vi "VI to JSON Graph Descr.vi"(8 "error in (no error)":errorcluster, 11 "vi path":path) -> (0 "error out":errorcluster, 2 "VI Description":string, 3 "JSON VI Graph":string)   [LabVIEW 2020]
doc: "**vi to json graph descrp.vi** scans recursivly a VI's Block Diagram\n(including nested structures such as Loops and Case Structures) and returns a JSON object describing all objects, their wiring, and constant values. Output has four top-level array keys:\n\n\"0\" — Objects\n Every GObject found on the diagram: nodes, terminals, wires, diagrams,\n structures, constants.\n Fields: ClassID (LabVIEW internal class ID), UID (unique ref ID, valid\n for this scan only), ClassName (e.g. \"Function\", \"Wire\", \"Terminal\",\n \"ForLoop\", \"DigitalNumericConstant\"), LabelText (visible caption, if\n any), OwnerClass / OwnerName / Ownder_UID (immediate parent GObject).\n Note: \"Ownder_UID\" is a known typo in the field name, kept as-is for\n compatibility — do not treat it as an error.\n\n\"1\" — Wires (node-level)\n One entry per wire. UID_Wire (matches a \"Wire\" Object in array 0),\n UID_Source (owning-node UID of the wire's source terminal), UIDs_Sink\n (owning-node UID(s) of its sink terminal(s)). A wire may branch to\n multiple sinks; the same node UID can appear more than once if several\n of its terminals are fed by the same wire.\n\n\"2\" — Terminal-Wire mapping\n Resolves array \"1\" down to the exact terminal. Fields: \"Terminal UID\"\n (matches a Terminal-class Object in array 0), \"Wire UID\", \"Caption\"\n (the terminal's visible name/role, e.g. \"x\", \"output cluster\", \"x+1\";\n empty if the terminal has no visible caption).\n\n\"3\" — Constant values\n Fields: \"Constant UID\" (matches a *Constant-class Object in array 0),\n \"Value String\" (the constant's value as a JSON-formatted string). For\n ClusterConstant this is a full nested JSON object of all its fields.\n\nResolving a wire to its exact source/sink terminals:\n 1. Look up the wire in array \"1\" ? UID_Source, UIDs_Sink (node-level).\n 2. Find all entries in array \"2\" with matching \"Wire UID\" ? candidate\n terminal UIDs.\n 3. For each candidate, look up its Ownder_UID in array \"0\": if it\n equals UID_Source, that terminal is the source; if it appears in\n UIDs_Sink, it is a sink terminal.\n 4. Use \"Caption\" from array \"2\" for the terminal's semantic role\n (cluster field name, parameter name, etc.).\n\nKnown limitations:\n - Duplicate object entries may occasionally appear for the same UID\n (root cause not yet identified).\n - ClusterConstant \"Value String\" duplicates the values of its child\n constants (also listed individually) — provided as a convenience\n aggregate, not an independent value.\n - A constant's LabelText is a free-form caption; it is not necessarily\n related to the terminal/field it feeds."
uses:
  <vilib>/Utility/traverseref.llb/TRef TravTarget.ctl
  ObjDescription.ctl
  Value of Constant.ctl
  Terminal and Wire.ctl
  Wire_Source_and_Sinks_IDs.ctl
  <vilib>/Utility/traverseref.llb/VI Scripting - Traverse.lvlib
  <vilib>/JDP Science/JSONtext/JSONtext.lvlib
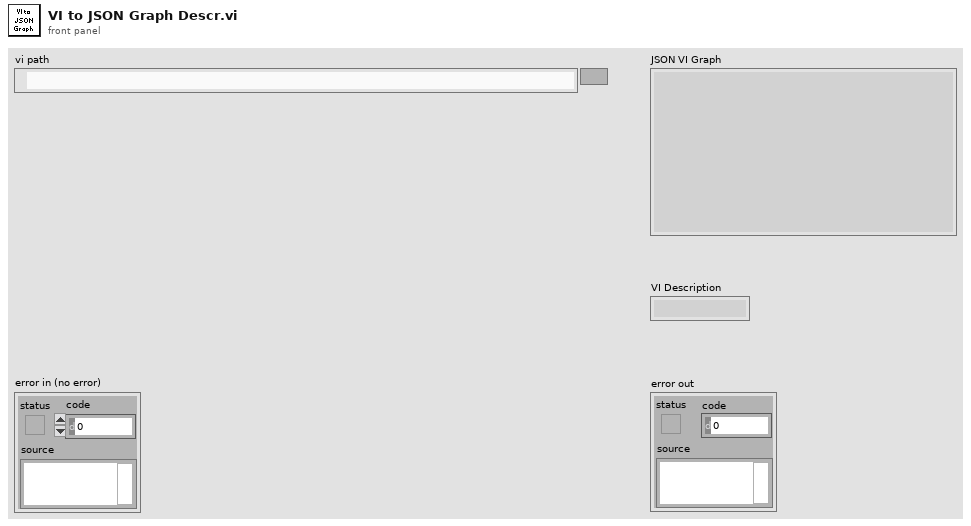
[diagram p1: front panel]
types:
  T1 = typedef "TRef TravTarget.ctl" = enum16{"FP", "BD", "Other"}
  T2 = typedef "ObjDescription.ctl" = cluster{"ClassID":u32, "UID":u32, "ClassName":string, "LabelText":string, "OwnerClass":string, "OwnerName":string, "Ownder_UID":u32}
  T3 = typedef "Value of Constant.ctl" = cluster{"Constant UID":i32, "Value String":string}
  T4 = typedef "Wire_Source_and_Sinks_IDs.ctl" = cluster{"UID_Wire":i32, "UID_Source":i32, "UIDs_Sink":i32[]}
  T5 = typedef "Terminal and Wire.ctl" = cluster{"Terminal UID":i32, "Wire UID":i32, "Caption":string}
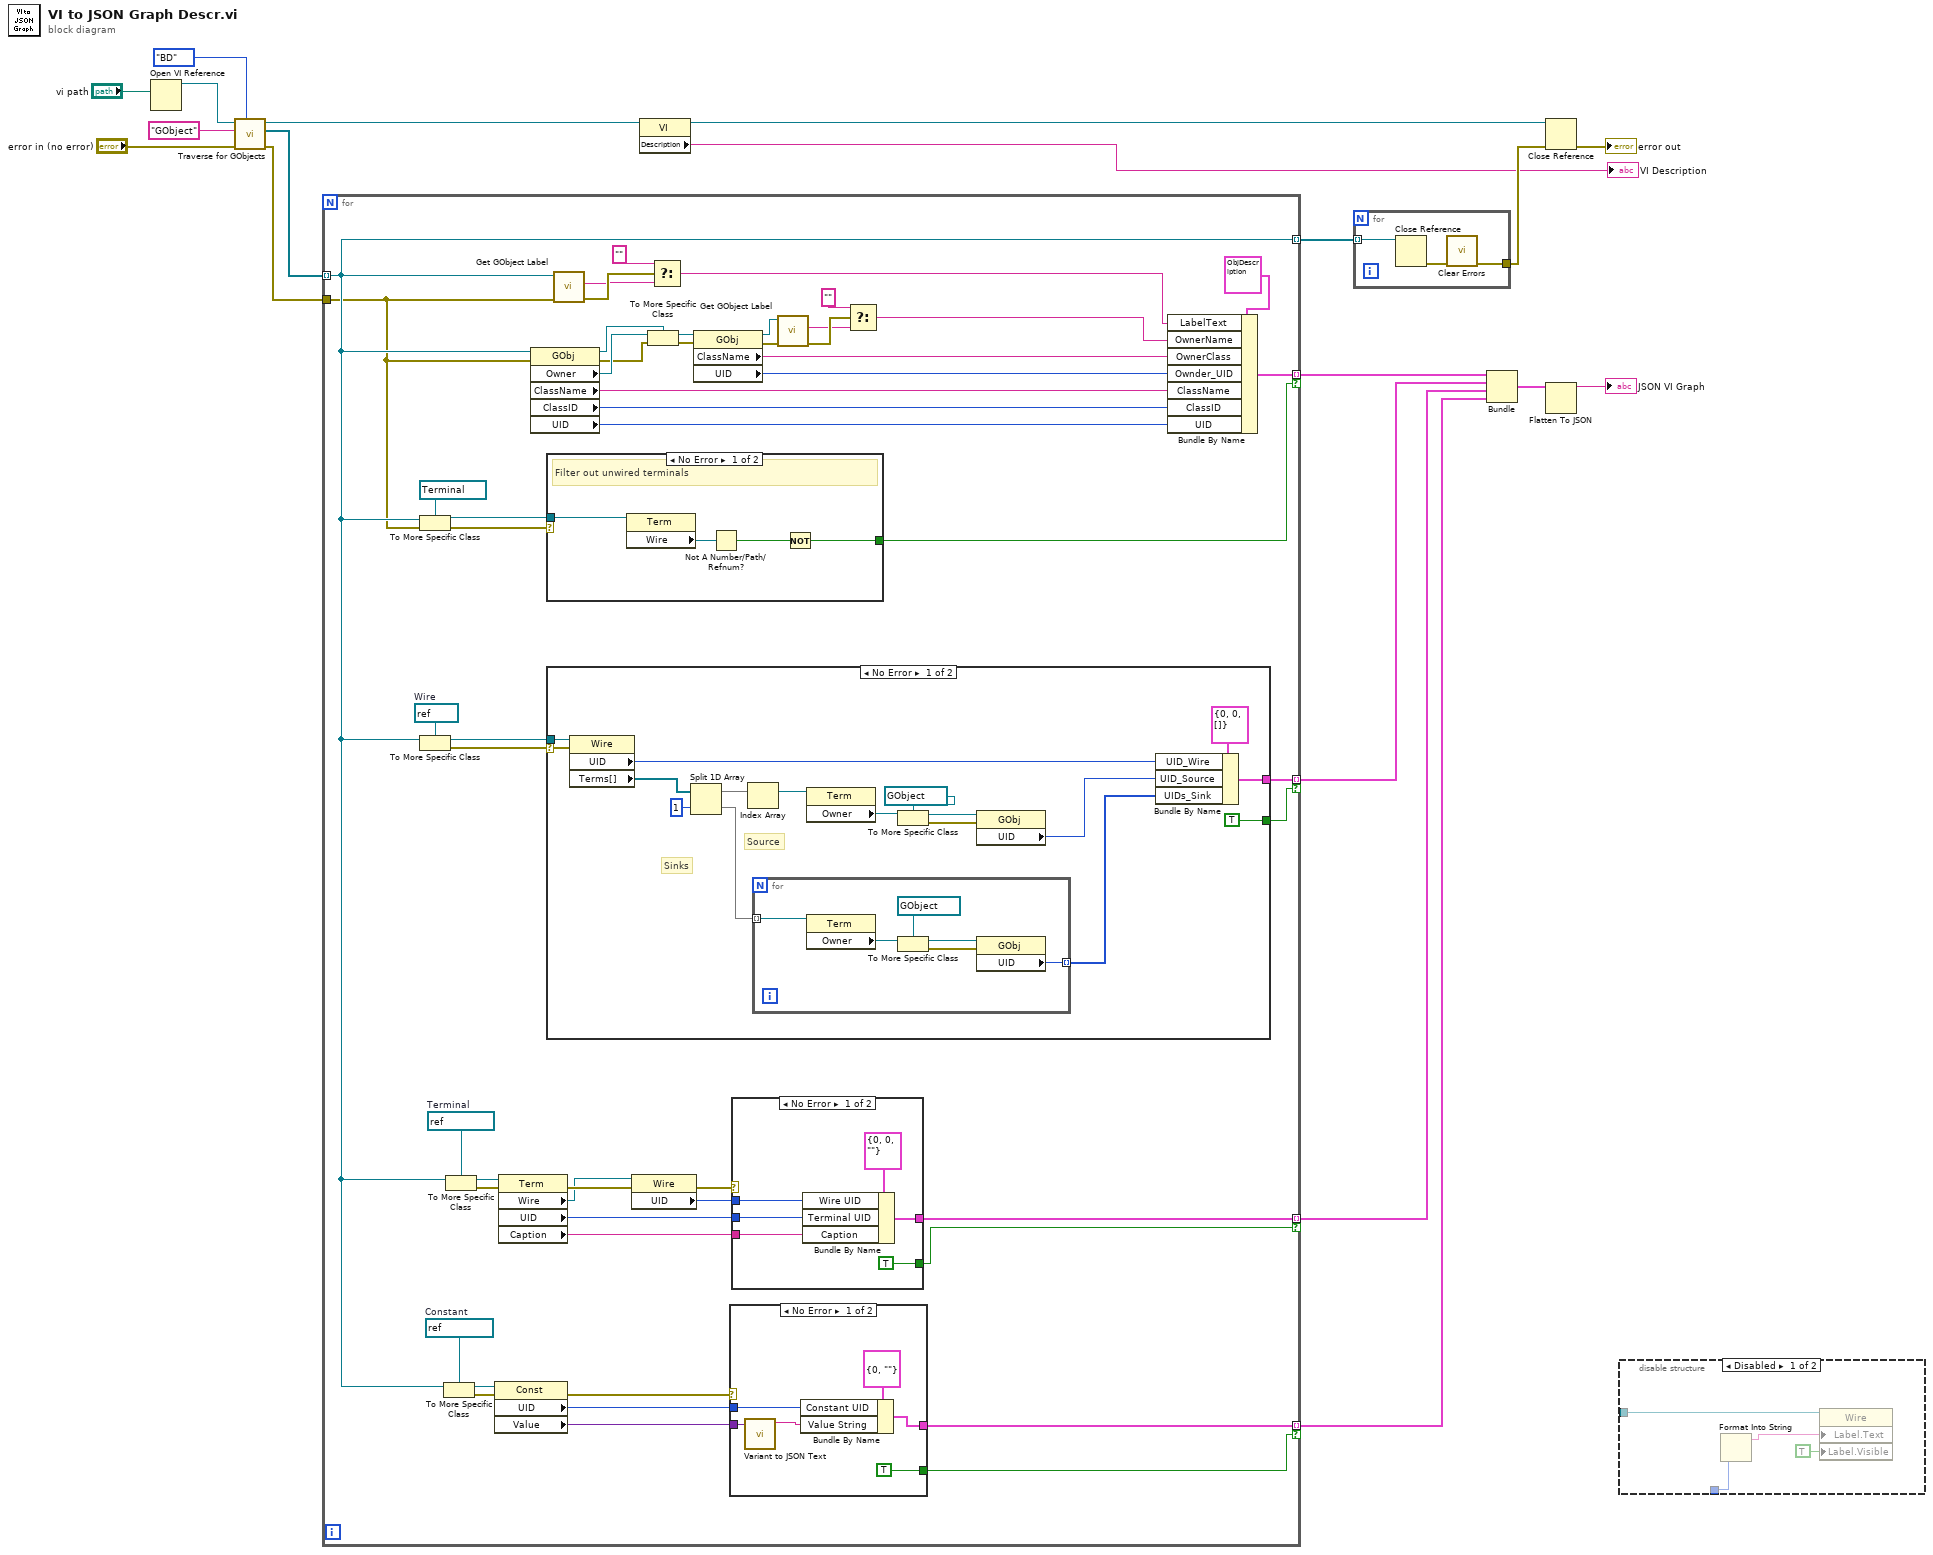
[diagram p0: block diagram]
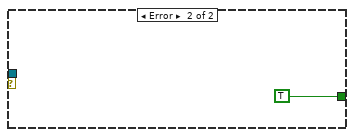
[diagram p2: hidden frame]
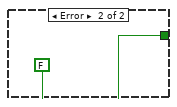
[diagram p4: hidden frame]
diagram:
  n1 = Open VI Reference(vi path="vi path") -> (vi reference=w17:refnum<vi>)  [unwired: 5 in, 1 out]
  n2 = call <vilib>:"Traverse for GObjects.vi"("Traverse Target"=TRef_TravTarget."BD", "error in (no error)"="error in (no error)", "Class Name"="GObject", "VI Refnum"=w17) -> ("error out"=w12:errorcluster, "References"=w19:refnum<vi>[], "dup VI Refnum"=w3:refnum<vi>)  [unwired: 4 in, 1 out]
  n3 = for {
    tunnel: w19 -> [w25] mode=indexing
    tunnel: [w66] -> w8 mode=indexing if=w20
    tunnel: [w25] -> w13 mode=indexing
    tunnel: w12 -> [w22]
    tunnel: [w46] -> w9 mode=indexing if=w45
    tunnel: [w43] -> w6 mode=indexing if=w42
    tunnel: [w27] -> w4 mode=indexing if=w26
    w30 = refnum<vi> refnum  # Constant
    w44 = refnum<vi> refnum  # Terminal
    w52 = refnum<vi> refnum  # Wire
    n4 = To More Specific Class(target class=refnum<vi> refnum ("reference out"), reference=w25, error in=w22) -> (specific class reference=w23:refnum<vi>, error out=w21:errorcluster)
    n5 = To More Specific Class(target class=w52, reference=w25) -> (specific class reference=w51:refnum<vi>, error out=w50:errorcluster)  [unwired: 1 in]
    n6 = To More Specific Class(target class=w30, reference=w25) -> (specific class reference=w31:refnum<vi>, error out=w32:errorcluster)  [unwired: 1 in]
    n7 = To More Specific Class(target class=w44, reference=w25) -> (specific class reference=w41:refnum<vi>, error out=w39:errorcluster)  [unwired: 1 in]
    n8 = property class="Const"(reference=w31, error in=w32) -> (error out=w33:errorcluster, "UID"=w28:i32, "Value"=w29:variant)  [unwired: 1 out]
    n9 = property class="Term"(reference=w41, error in=w39) -> (error out=w38:errorcluster, "Wire"=w35:refnum<vi>, "UID"=w34:i32, "Caption"=w36:string)  [unwired: 1 out]
    n10 = property class="GObj"(reference=w25, error in=w22) -> (reference out=w53:refnum<vi>, error out=w57:errorcluster, "Owner"=w69:refnum<vi>, "ClassName"=w48:string, "ClassID"=w47:u32, "UID"=w55:i32)
    n11 = case shown="No Error" w21 {
      tunnel: w23 -> [w75 _]
      tunnel: [w72 TRUE] -> w20
      frame No Error {
        # "Filter out unwired terminals"
        n12 = property class="Term"(reference=w75) -> ("Wire"=w74:refnum<vi>)  [unwired: 1 in, 2 out]
        n13 = Not A Number/Path/Refnum?(number/path/refnum=w74) -> (NaN/Path/Refnum?=w73:bool)
        n14 = Not(x=w73) -> (.not. x?=w72:bool)
      }
      frame Error {
      }
    }
    n15 = case shown="No Error" w50 {
      selector: w50 -> [w98 _]
      tunnel: w51 -> [w99 _]
      tunnel: [w89 _] -> w46
      tunnel: [TRUE FALSE] -> w45
      frame No Error {
        # "Sinks"
        # "Source"
        n16 = property class="Wire"(reference=w99, error in=w98) -> ("UID"=w83:i32, "Terms[]"=w87:refnum<vi>[])  [unwired: 2 out]
        n17 = Split 1D Array(array=w87, index=1 ("length")) -> (first subarray=w95:refnum<vi>[], second subarray=w94:refnum<vi>[])
        n18 = Index Array(array=w95) -> (element=w96:refnum<vi>)  [unwired: 1 in]
        n19 = for {
          tunnel: w94 -> [w105] mode=indexing
          tunnel: [w100] -> w84 mode=indexing
          n20 = property class="Term"(reference=w105) -> ("Owner"=w101:refnum<vi>)  [unwired: 1 in, 2 out]
          n21 = To More Specific Class(target class=refnum<vi> refnum ("reference out"), reference=w101) -> (specific class reference=w103:refnum<vi>, error out=w102:errorcluster)  [unwired: 1 in]
          n22 = property class="GObj"(reference=w103, error in=w102) -> ("UID"=w100:i32)  [unwired: 2 out]
        }
        n23 = property class="Term"(reference=w96) -> ("Owner"=w91:refnum<vi>)  [unwired: 1 in, 2 out]
        n24 = To More Specific Class(target class=refnum<vi> refnum ("reference out"), reference=w91) -> (specific class reference=w92:refnum<vi>, error out=w93:errorcluster)  [unwired: 1 in]
        n25 = property class="GObj"(reference=w92, error in=w93) -> ("UID"=w85:i32)  [unwired: 2 out]
        n26 = Bundle By Name(cluster=T4 {"UID_Wire"=0, "UID_Source"=0, "UIDs_Sink"=[]} ("output cluster"), "UID_Wire"=w83, "UID_Source"=w85, "UIDs_Sink"=w84) -> (w89:T4)
      }
      frame Error {
      }
    }
    n27 = call <vilib>:"Get GObject Label.vi"("error in (no error)"=w22, "GObject"=w25) -> ("error out"=w70:errorcluster, "Object Label"=w68:string)  [unwired: 5 in, 3 out]
    n28 = property class="Wire"(reference=w35, error in=w38) -> (error out=w37:errorcluster, "UID"=w40:i32)  [unwired: 1 out]
    n29 = To More Specific Class(target class=w53, reference=w69, error in=w57) -> (specific class reference=w61:refnum<vi>, error out=w56:errorcluster)
    n30 = Select(t="", s=w70, f=w68) -> (s? t:f=w49:string)
    n31 = property class="GObj"(reference=w61, error in=w56) -> (reference out=w60:refnum<vi>, error out=w58:errorcluster, "ClassName"=w54:string, "UID"=w59:i32)
    n32 = case shown="No Error" w33 {
      tunnel: [TRUE _] -> w26
      tunnel: [w81 _] -> w27
      tunnel: w29 -> [w78 _]
      tunnel: w28 -> [w79 _]
      frame No Error {
        n33 = call <vilib>:"Variant to JSON Text.vi"("Variant"=w78) -> ("<JSON>"=w77:string)  [unwired: 8 in, 2 out]
        n34 = Bundle By Name(cluster=T3 {"Constant UID"=0, "Value String"=""} ("Terminal and wire"), "Constant UID"=w79, "Value String"=w77) -> (w81:T3)
      }
      frame Error {
      }
    }
    n35 = case shown="No Error" w37 {
      tunnel: [TRUE _] -> w42
      tunnel: [w111 _] -> w43
      tunnel: w40 -> [w107 _]
      tunnel: w36 -> [w109 _]
      tunnel: w34 -> [w108 _]
      frame No Error {
        n36 = Bundle By Name(cluster=T5 {"Terminal UID"=0, "Wire UID"=0, "Caption"=""} ("output cluster"), "Wire UID"=w107, "Terminal UID"=w108, "Caption"=w109) -> (w111:T5)
      }
      frame Error {
      }
    }
    n37 = call <vilib>:"Get GObject Label.vi"("error in (no error)"=w58, "GObject"=w60) -> ("error out"=w71:errorcluster, "Object Label"=w63:string)  [unwired: 5 in, 3 out]
    n38 = Select(t="", s=w71, f=w63) -> (s? t:f=w62:string)
    n39 = Bundle By Name(cluster=T2 {"ClassID"=16395, "UID"=16395, "ClassName"="ControlTerminal", "LabelText"="ControlTerminal", "OwnerClass"="Owner Obj Class", "OwnerName"="Owner Obj Label", "Ownder_UID"=16395} ("Cluster"), "LabelText"=w49, "OwnerName"=w62, "OwnerClass"=w54, "Ownder_UID"=w59, "ClassName"=w48, "ClassID"=w47, "UID"=w55) -> (w66:T2)
  }
  n40 = property class="VI"(reference=w3) -> (reference out=w2:refnum<vi>, "Description"=→"VI Description":string)  [unwired: 1 in, 1 out]
  n41 = for {
    tunnel: w13 -> [w115] mode=indexing
    tunnel: [w113] -> w11
    n42 = Close Reference(reference=w115) -> (error out=w114:errorcluster)  [unwired: 1 in]
    n43 = call <vilib>:"Clear Errors.vi"("error in (no error)"=w114) -> ("error out"=w113:errorcluster)  [unwired: 5 in, 1 out]
  }
  n44 = Bundle(w8, w9, w6, w4) -> (w5:cluster{T2[], T4[], T5[], T3[]})  [unwired: 1 in]
  n45 = Close Reference(reference=w2, error in (no error)=w11) -> (error out=→"error out":errorcluster)
  n46 = Flatten To JSON(anything=w5) -> (JSON string=→"JSON VI Graph":string)  [unwired: 2 in, 1 out]
  n47 = disable-structure shown="Disabled" {
    disable-tunnel: _ -> [w119 _]
    disable-tunnel: _ -> [w118 _]
    frame Disabled {
      n48 = Format Into String(w118) -> (resulting string=w117:string)  [unwired: 3 in, 1 out]
      n49 = property class="Wire"(reference=w119, "Label.Text"=w117, "Label.Visible"=TRUE) -> ()  [unwired: 1 in, 2 out]
    }
    frame Enabled {
    }
  }
